vi "Start Sync.vi"(8 "error in (no error)":errorcluster, 11 "gRPC Server in":refnum<class "RouteGuide.lvclass">) -> (0 "error out":errorcluster, 3 "gRPC Server out":refnum<class "RouteGuide.lvclass">)   [LabVIEW 2019, in "route_guide_server.lvlib" / "RouteGuide.lvclass"]
uses:
  RouteGuide.lvclass
  RPC Messages/routeguide_Point.ctl
  route_guide_server.lvlib
  RPC Messages/routeguide_Feature.ctl
  <vilib>/gRPC/LabVIEW gRPC Library/gprc-lvsupport-release.lvlib
  RPC Messages/routeguide_RouteSummary.ctl
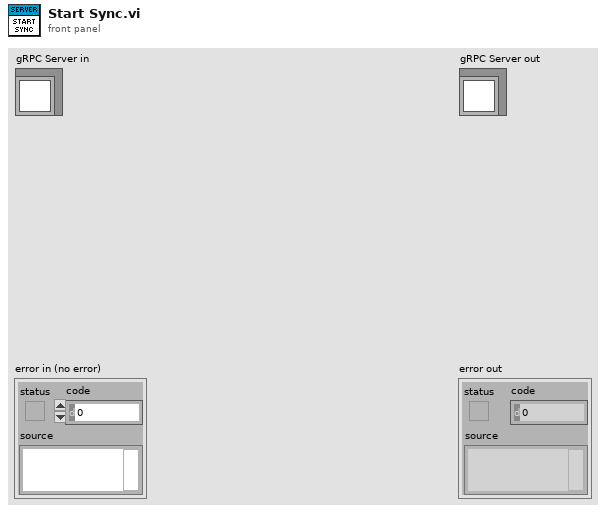
[diagram p1: front panel]
types:
  T1 = typedef "route_guide_server.lvlib/routeguide_Feature.ctl" = cluster{"name":string, "location":T2}
  T2 = typedef "route_guide_server.lvlib/routeguide_Point.ctl" = cluster{"latitude":i32, "longitude":i32}
  T3 = typedef "route_guide_server.lvlib/routeguide_RouteSummary.ctl" = cluster{"point_count":i32, "feature_count":i32, "distance":i32, "elapsed_time":i32}
  T4 = typedef "route_guide_server.lvlib/RouteGuide.lvclass/Server Internal UEs.ctl" = cluster{"routeguide_RouteGuide_GetFeature Internal UE":refnum<user-event>, "routeguide_RouteGuide_ListFeatures Internal UE":refnum<user-event>, "routeguide_RouteGuide_RecordRoute Internal UE":refnum<user-event>, "routeguide_RouteGuide_RouteChat Internal UE":refnum<user-event>}
  T5 = typedef "route_guide_server.lvlib/RouteGuide.lvclass/Server gRPC UEs.ctl" = cluster{"routeguide_RouteGuide_GetFeature gRPC UE":refnum<user-event>, "routeguide_RouteGuide_ListFeatures gRPC UE":refnum<user-event>, "routeguide_RouteGuide_RecordRoute gRPC UE":refnum<user-event>, "routeguide_RouteGuide_RouteChat gRPC UE":refnum<user-event>}
  T6 = typedef "gprc-lvsupport-release.lvlib/grpcId.ctl" = u64
  T7 = typedef "route_guide_server.lvlib/routeguide_Rectangle.ctl" = cluster{"lo":T2, "hi":T2}
  T8 = typedef "route_guide_server.lvlib/routeguide_RouteNote.ctl" = cluster{"location":T2, "message":string}
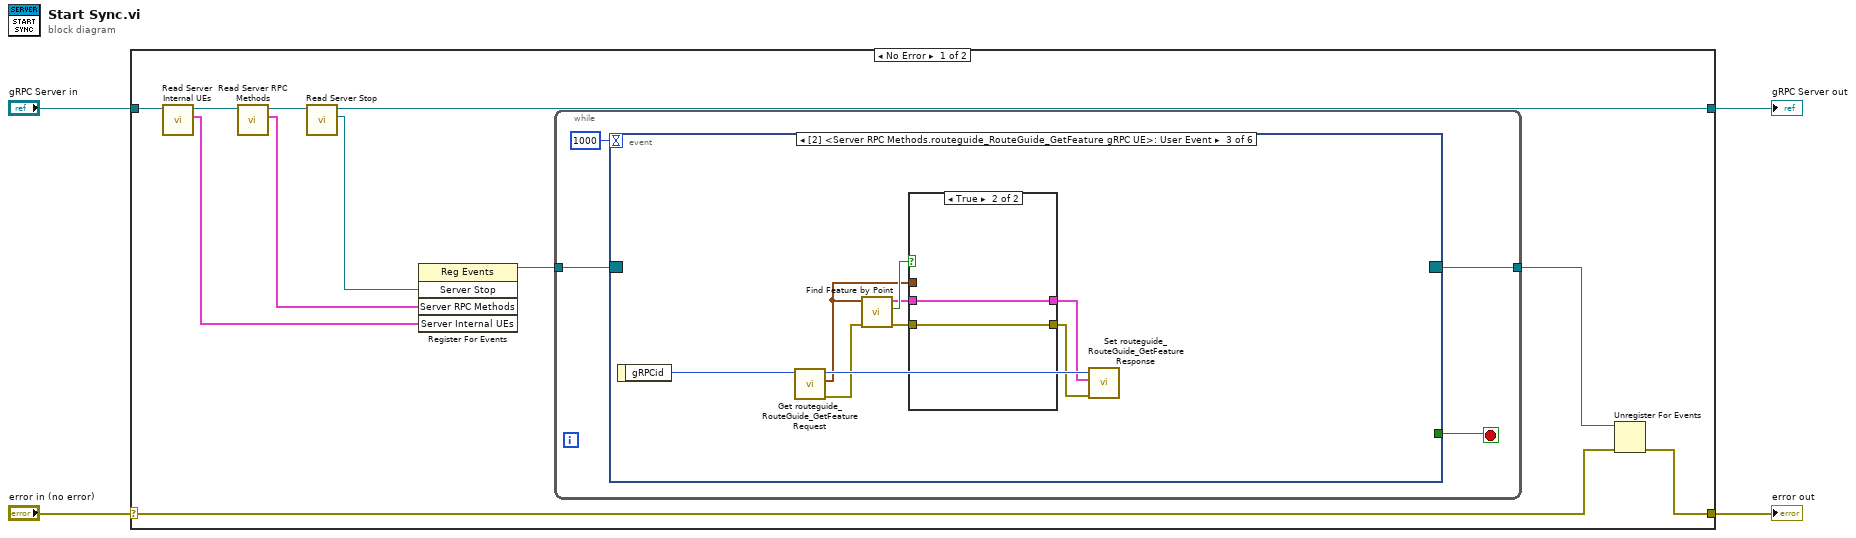
[diagram p0: block diagram]
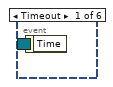
[diagram p2: hidden frame]
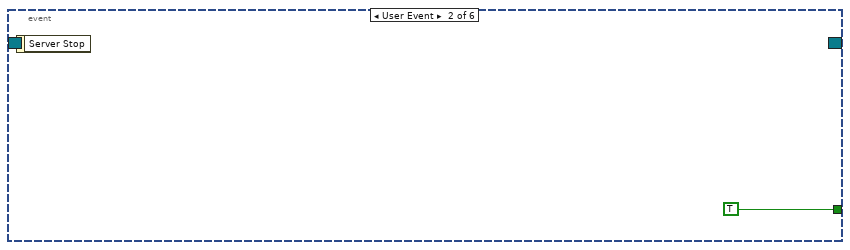
[diagram p3: hidden frame]
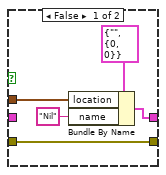
[diagram p4: hidden frame]
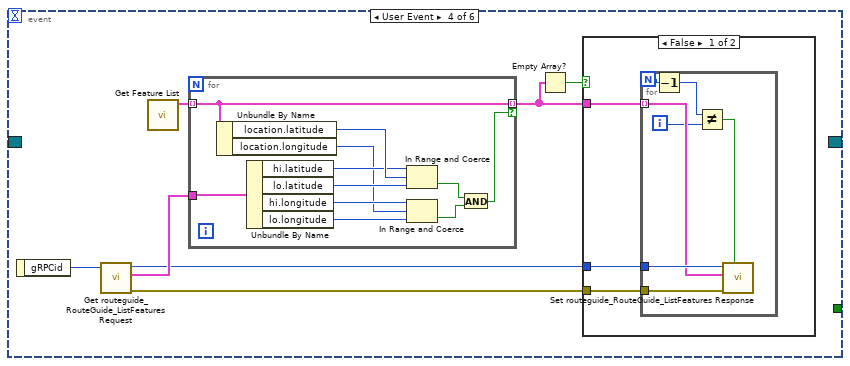
[diagram p5: hidden frame]
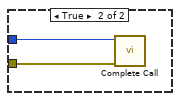
[diagram p6: hidden frame]
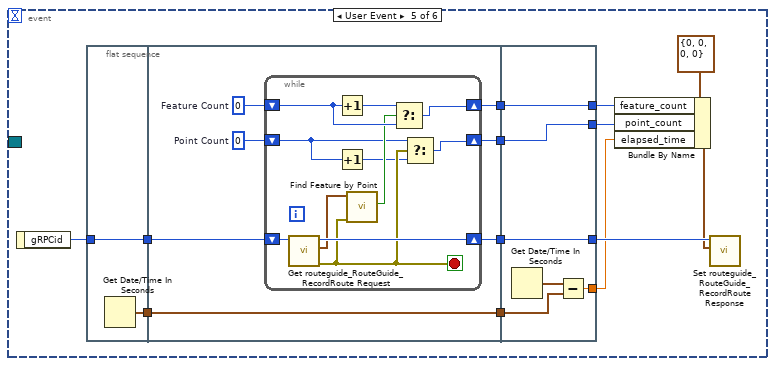
[diagram p7: hidden frame]
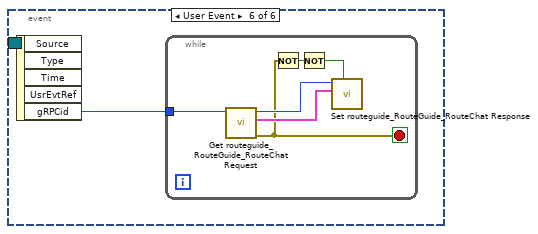
[diagram p8: hidden frame]
diagram:
  n1 = case shown="No Error" "error in (no error)" {
    selector: "error in (no error)" -> [w9 w114]
    tunnel: [w8 w114] -> w3
    tunnel: [w6 w113] -> w1
    tunnel: "gRPC Server in" -> [w15 w113]
    frame No Error {
      n2 = call "Read Server Internal UEs.vi"("SignalGeneratorService in"=w15) -> ("Server Internal UEs"=w13:T4, "SignalGeneratorService out"=w14:refnum<class "RouteGuide.lvclass">)  [unwired: 8 in, 1 out]
      n3 = call "Read Server RPC Methods.vi"("SignalGeneratorService in"=w14) -> ("Server RPC Methods"=w7:T5, "SignalGeneratorService out"=w12:refnum<class "RouteGuide.lvclass">)  [unwired: 8 in, 1 out]
      n4 = call-dynamic "Read Server Stop.vi"("iService in"=w12) -> ("Server Stop"=w5:refnum<user-event>, "iService out"=w6:refnum<class "RouteGuide.lvclass">)  [unwired: 8 in, 1 out]
      n5 = register-events(w5, w7, w13) -> (reference out=w11:refnum<event-registration>)  [unwired: 2 in, 1 out]
      n6 = while {
        tunnel: w11 -> [w19]
        tunnel: [w17] -> w10
        stop <- w18 stop-if-true
        n7 = event "RPC Methods Event Structure" shown="[2] <Server RPC Methods.routeguide_RouteGuide_GetFeature gRPC UE>: User Event" {
          selector: w19 -> [_ _ _ _ _ _]
          dyn-events: [_ _ _ _ _ _] -> w17
          timeout: 1000 -> [_ _ _ _ _ _]
          tunnel: [_ TRUE _ _ _ _] -> w18
          event Timeout {
            n8 = event-data() -> ()  [unwired: 1 in, 1 out]
          }
          event User Event {
            n9 = event-data() -> ()  [unwired: 1 in, 1 out]
          }
          event User Event {
            n10 = event-data() -> ("gRPCid"=w29:T6)  [unwired: 1 in]
            n11 = call "Get routeguide_RouteGuide_GetFeature Request.vi"("gRPCid in"=w29) -> ("error out"=w27:errorcluster, "Message Data"=w21:T2, "gRPCid out"=w28:T6)  [unwired: 8 in]
            n12 = call "Find Feature by Point.vi"("error in"=w27, "Point"=w21) -> ("error out"=w24:errorcluster, "Found?"=w26:bool, "Feature"=w25:cluster{"name":string, "location":T2})  [unwired: 7 in]
            n13 = case shown="True" w26 {
              tunnel: w25 -> [_ w36]
              tunnel: w24 -> [w34 w35]
              tunnel: [w32 w36] -> w23
              tunnel: [w34 w35] -> w22
              tunnel: w21 -> [w31 _]
              frame False {
                n14 = Bundle By Name(cluster=T1 {"name"="", "location"={"latitude"=0, "longitude"=0}} ("Message Data"), "location"=w31, "name"="Nil") -> (w32:T1)
              }
              frame True {
              }
            }
            n15 = call "Set routeguide_RouteGuide_GetFeature Response.vi"("error in (no error)"=w22, "Message Data"=w23, "gRPCid in"=w28) -> ()  [unwired: 8 in, 1 out]
          }
          event User Event {
            n16 = event-data() -> ("gRPCid"=w43:T6)  [unwired: 1 in]
            n17 = call "Get routeguide_RouteGuide_ListFeatures Request.vi"("gRPCid in"=w43) -> ("error out"=w39:errorcluster, "Message Data"=w41:T7, "gRPCid out"=w40:T6)  [unwired: 8 in]
            n18 = call "Get Feature List.vi"() -> ("Feature List"=w42:cluster{"name":string, "location":T2}[])  [unwired: 10 in, 1 out]
            n19 = for {
              tunnel: w42 -> [w57] mode=indexing
              tunnel: w41 -> [w66]
              tunnel: [w57] -> w37 mode=indexing if=w56
              n20 = Unbundle By Name(w57) -> ("location.latitude"=w65:i32, "location.longitude"=w60:i32)
              n21 = Unbundle By Name(w66) -> ("hi.latitude"=w64:i32, "lo.latitude"=w63:i32, "hi.longitude"=w62:i32, "lo.longitude"=w61:i32)
              n22 = In Range and Coerce(upper limit=w64, x=w65, lower limit=w63) -> (In Range?=w58:bool)  [unwired: 1 out]
              n23 = In Range and Coerce(upper limit=w62, x=w60, lower limit=w61) -> (In Range?=w59:bool)  [unwired: 1 out]
              n24 = And(x=w58, y=w59) -> (x .and. y?=w56:bool)
            }
            n25 = Empty Array?(array=w37) -> (empty?=w38:bool)
            n26 = case shown="False" w38 {
              tunnel: w40 -> [w46 w54]
              tunnel: w39 -> [w45 w55]
              tunnel: w37 -> [w44 _]
              frame False {
                n27 = for {
                  N -> [w50]
                  tunnel: w46 -> [w53]
                  tunnel: w45 -> [w52]
                  tunnel: w44 -> [w51] mode=indexing
                  i -> [w49]
                  n28 = Decrement(x=w50) -> (x-1=w48:i32)
                  n29 = Not Equal?(x=w48, y=w49) -> (x != y?=w47:bool)
                  n30 = call "Set routeguide_RouteGuide_ListFeatures Response.vi"("Streeming? (F)"=w47, "error in (no error)"=w52, "Message Data"=w51, "gRPCid in"=w53) -> ()  [unwired: 7 in, 1 out]
                }
              }
              frame True {
                n31 = call <vilib>:"Complete Call.vi"("gRPCid"=w54, "error in (no error)"=w55) -> ()  [unwired: 8 in, 1 out]
              }
            }
          }
          event User Event {
            n32 = event-data() -> ("gRPCid"=w79:T6)  [unwired: 1 in]
            n33 = flat-sequence {
              tunnel: w79 -> [w81]
              tunnel: [w81] -> w74
              tunnel: [w80] -> w69
              tunnel: w74 -> [w88]
              tunnel: [w87] -> w73
              tunnel: [w82] -> w72
              tunnel: [w85] -> w71
              tunnel: w69 -> [w84]
              tunnel: [w84] -> w68
              tunnel: [w104] -> w76
              tunnel: [w105] -> w78
              tunnel: w73 -> [w105]
              tunnel: w72 -> [w104]
              tunnel: [w103] -> w70
              tunnel: w71 -> [w103]
              tunnel: w68 -> [w101]
              tunnel: [w100] -> w67
              frame #0 {
                n34 = Get Date/Time In Seconds() -> (seconds since 1Jan1904=w80:timestamp)
              }
              frame #1 {
                w83 = 0  # Point Count
                w86 = 0  # Feature Count
                n35 = while {
                  shift-right: [w98] -> w87
                  shift-left: w88 -> [w99]
                  shift-right: [w96] -> w85
                  shift-left: w86 -> [w95]
                  shift-right: [w92] -> w82
                  shift-left: w83 -> [w89]
                  stop <- w91 stop-if-true
                  n36 = call "Get routeguide_RouteGuide_RecordRoute Request.vi"("gRPCid in"=w99) -> ("error out"=w91:errorcluster, "Message Data"=w97:T2, "gRPCid out"=w98:T6)  [unwired: 8 in]
                  n37 = Increment(x=w95) -> (x+1=w94:i32)
                  n38 = Increment(x=w89) -> (x+1=w90:i32)
                  n39 = call "Find Feature by Point.vi"("error in"=w91, "Point"=w97) -> ("Found?"=w93:bool)  [unwired: 7 in, 2 out]
                  n40 = Select(t=w94, s=w93, f=w95) -> (s? t:f=w96:i32)
                  n41 = Select(t=w89, s=w91, f=w90) -> (s? t:f=w92:i32)
                }
              }
              frame #2 {
                n42 = Get Date/Time In Seconds() -> (seconds since 1Jan1904=w102:timestamp)
                n43 = Subtract(x=w102, y=w101) -> (x-y=w100:dbl)
              }
            }
            n44 = Bundle By Name(cluster=T3 {"point_count"=0, "feature_count"=0, "distance"=0, "elapsed_time"=0} ("Message Data"), "feature_count"=w70, "point_count"=w76, "elapsed_time"=w67) -> (w75:T3)
            n45 = call "Set routeguide_RouteGuide_RecordRoute Response.vi"("Message Data"=w75, "gRPCid in"=w78) -> ()  [unwired: 9 in, 1 out]
          }
          event User Event {
            n46 = event-data() -> ("gRPCid"=w106:T6)  [unwired: 1 in, 4 out]
            n47 = while {
              tunnel: w106 -> [w112]
              stop <- w109 stop-if-true
              n48 = call "Get routeguide_RouteGuide_RouteChat Request.vi"("gRPCid in"=w112) -> ("error out"=w109:errorcluster, "Message Data"=w110:T8, "gRPCid out"=w111:T6)  [unwired: 8 in]
              n49 = Not(x=w109) -> (.not. x?=w108:bool)
              n50 = Not(x=w108) -> (.not. x?=w107:bool)
              n51 = call "Set routeguide_RouteGuide_RouteChat Response.vi"("Streeming? (F)"=w107, "Message Data"=w110, "gRPCid in"=w111) -> ()  [unwired: 8 in, 1 out]
            }
          }
        }
      }
      n52 = Unregister For Events(event registration refnum=w10, error in=w9) -> (error out=w8:errorcluster)
    }
    frame Error {
    }
  }
  "error out" <- w3
  "gRPC Server out" <- w1
